vi "readFromXML.vi"(8 "error in (no error)":errorcluster, 10 "XML in":string, 11 "UpdateIERS in":refnum<class "UpdateIERS.lvclass">) -> (0 "error out":errorcluster, 3 "UpdateIERS out":refnum<class "UpdateIERS.lvclass">)   [LabVIEW 2022 SP3, in "TCSDataDefinitions.lvlib" / "TCSTimeComponentCommand.lvlib" / "UpdateIERS.lvclass"]
uses:
  UpdateIERS.lvclass
  TCSIersCommand/TCSIersCommand.lvclass
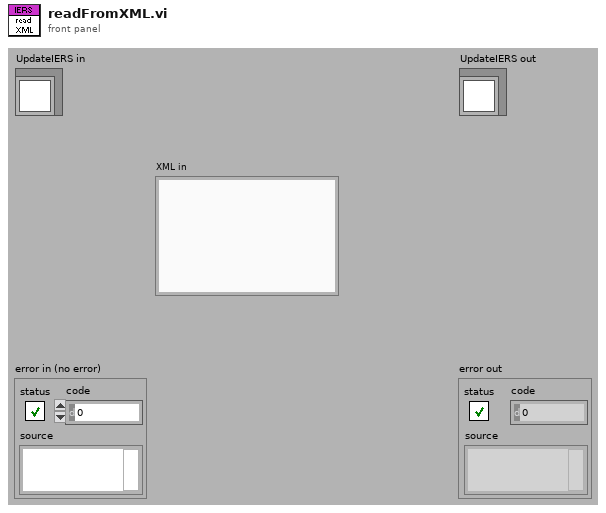
[diagram p1: front panel]
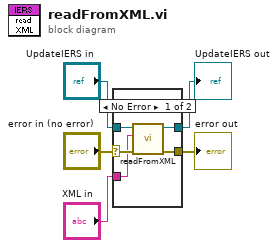
[diagram p0: block diagram]
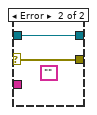
[diagram p2: hidden frame]
diagram:
  n1 = case shown="No Error" "error in (no error)" {
    selector: "error in (no error)" -> [w10 w12]
    tunnel: [w6 w12] -> w4
    tunnel: [w8 w11] -> w2
    tunnel: "UpdateIERS in" -> [w9 w11]
    tunnel: "XML in" -> [w7 _]
    frame No Error {
      n2 = call-parent "readFromXML.vi"("error in (no error)"=w10, "XMLin"=w7, "TCSIersCommand in"=w9) -> ("error out"=w6:errorcluster, "TCSIersCommand out"=w8:refnum<class "UpdateIERS.lvclass">)  [unwired: 7 out]
    }
    frame Error {
      (unwired) ""
    }
  }
  "error out" <- w4
  "UpdateIERS out" <- w2
